vi "Global 4.vi"() -> ()   [LabVIEW 2020]
panel:
  in  "Boolean":bool
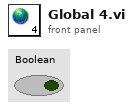
[diagram p1: front panel]
diagram:
